vi "Shutdown.vi"(8 "error in":errorcluster) -> (0 "error out":errorcluster)   [LabVIEW 2020, in "GUI.lvlib"]
uses:
  GUI.lvlib
  Eventing/Event FGV Actions.ctl
panel:
  # "Event Handler: Shutdown"
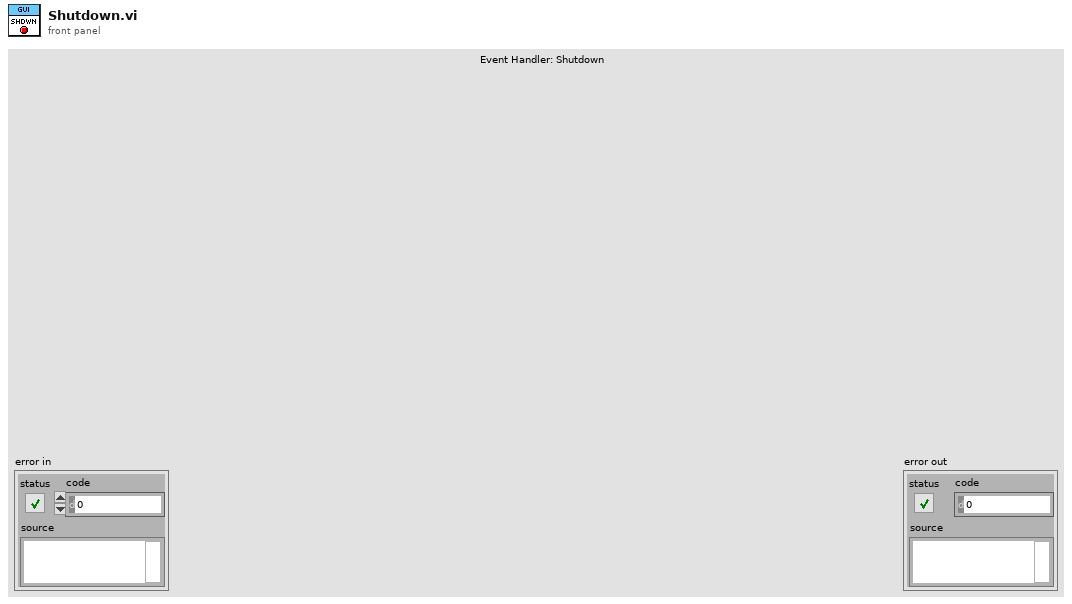
[diagram p1: front panel]
types:
  T1 = typedef "GUI.lvlib/Event FGV Actions.ctl" = enum16{"Get", "Create", "Destroy"}
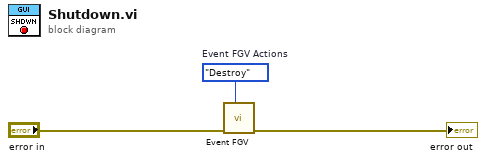
[diagram p0: block diagram]
diagram:
  w3 = Event_FGV_Actions."Destroy"  # Event FGV Actions
  n1 = call "Event FGV.vi"("Event FGV Actions"=w3, "error in"="error in") -> ("error out"=→"error out":errorcluster)  [unwired: 7 in, 2 out]
